vi "Set Boolean.vi"(8 "error in (no error)":errorcluster, 10 "Boolean":bool, 11 "ByRef Example in":refnum<class "ByRef Example.lvclass">) -> (0 "error out":errorcluster, 3 "ByRef Example out":refnum<class "ByRef Example.lvclass">)   [LabVIEW 2012, in "ByRef Example.lvclass"]
uses:
  ByRef Example.lvclass
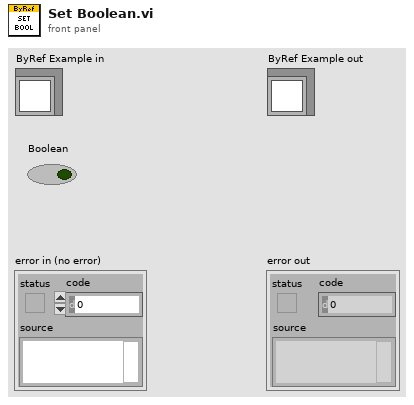
[diagram p1: front panel]
types:
  T1 = typedef "ByRef Example.lvclass/Ref Data.ctl" = cluster{"Boolean":bool, "Numeric":dbl, "String":string}
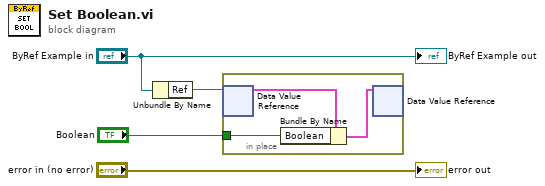
[diagram p0: block diagram]
diagram:
  n1 = Unbundle By Name("ByRef Example in") -> ("Ref"=w3:refnum<data-value>)
  n2 = in-place {
    in-place-border: "Boolean" -> [w5]
    n3 = in-place-dvr #1(w3) -> (w7:T1)  [unwired: 1 out]
    n4 = Bundle By Name(cluster=w7, "Boolean"=w5) -> (w6:T1)
    n5 = in-place-dvr #1(w6) -> ()  [unwired: 2 out]
  }
  "error out" <- "error in (no error)"
  "ByRef Example out" <- "ByRef Example in"
